vi "GEOM_GetReadModes.vi"() -> (2 "readmodes":string[](array[string]))   [LabVIEW 2016]
uses:
  GEOM_VAR_action.ctl
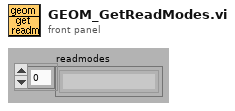
[diagram p1: front panel]
types:
  T1 = typedef "GEOM_VAR_action.ctl" = enum16{"read", "write"}
  T2 = typedef "GEOM_FPAReadMode.ctl" = cluster{"name":string, "Amplifiers":T3[]}
  T3 = typedef "GEOM_Amplifier.ctl" = cluster{"number":i32, "type":T4, "rotated":i16, "fliped":u16, "FPAcoord":cluster{"xstart":i32, "ystart":i32}, "Physical_size":cluster{"columns":i32, "rows":i32}, "predata":cluster{"columns":i32, "rows":i32}, "postdata":cluster{"columns":i32, "rows":i32}, "Req ROIs":T5, "Corr ROI":T5, "Detnumber":i32, "ampID":string, "discard":i32}
  T4 = typedef "GEOM_AmpType.ctl" = u16
  T5 = typedef "GEOM_ROI.ctl" = T6[]
  T6 = typedef "GEOM_Coords.ctl" = cluster{"xstart":u32, "ystart":u32, "xsize":u32, "ysize":u32}
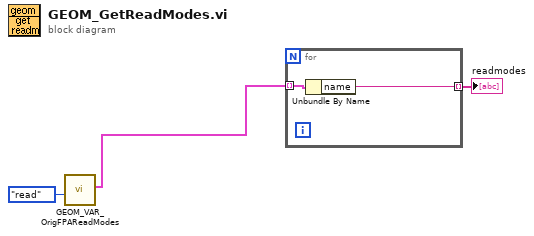
[diagram p0: block diagram]
diagram:
  n1 = call "GEOM_VAR_OrigFPAReadModes.vi"("Action"=GEOM_VAR_action."read") -> ("GEOM_OrigFPAReadModes out"=w2:T2[])  [unwired: 1 in, 9 out]
  n2 = for {
    tunnel: w2 -> [w5] mode=indexing
    tunnel: [w4] -> w3 mode=indexing
    n3 = Unbundle By Name(w5) -> ("name"=w4:string)
  }
  "readmodes" <- w3
